vi "ArrayBuilder.vi"(10 "data":dynamicdata(waveform)) -> (3 "Array":dbl[][](array[numeric]))   [LabVIEW 2011]
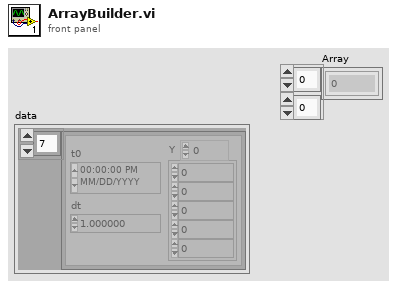
[diagram p1: front panel]
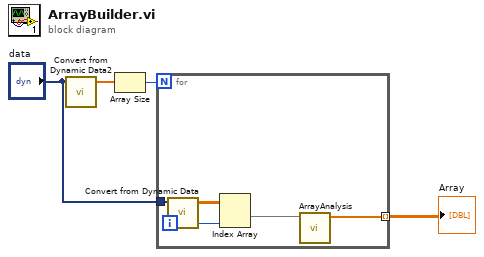
[diagram p0: block diagram]
diagram:
  n1 = call "Convert from Dynamic Data2"("Dynamic Data Type"="data") -> ("Array"=w1:dbl[])  [unwired: 3 in]
  n2 = Array Size(array=w1) -> (size(s)=w2:i32)
  n3 = for {
    N: w2 -> [_]
    tunnel: "data" -> [w9]
    tunnel: [w5] -> w4 mode=indexing
    i -> [w7]
    n4 = call "Convert from Dynamic Data"("Dynamic Data Type"=w9) -> ("Array"=w8:dbl[][])  [unwired: 3 in]
    n5 = Index Array "Index Array"(array=w8, index (col)=w7) -> (element=w6:dbl[])  [unwired: 1 in]
    n6 = call "ArrayAnalysis.vi"("Array in"=w6) -> ("Array out"=w5:dbl[])  [unwired: 10 in]
  }
  "Array" <- w4
